vi "PicoScopeospaExampleAWG.vi"() -> ()   [LabVIEW 2010]
uses:
  psospa.dll
panel:
  in  "General AWG Settings":T1={"Peak-to-Peak Voltage"=2.0, "Offset Voltage"=0.0, "Wave Type"=17, "Sweep Type"=0, "Cycles"=10, "Trigger Type"=0, "Trigger Source"=4, "sigGenEnabled"=TRUE, "Trigger Enabled"=FALSE, "autoTriggerPicoSeconds"=0} {"Trigger Source" items=["None"=0, "Scope Trigger"=1, "Software Trigger"=4, "Trigger Raw"=5]; "Trigger Type" items=["Rising", "Falling", "Gate High", "Gate Low"]; "Sweep Type" items=["Up", "Down", "Up-Down", "Down-Up"]; "Wave Type" items=["Sine"=17, "Square"=18, "Triangle"=19, "Ramp Up"=20, "Ramp Down"=21, "Sinc"=22, "Gaussian"=23, "Half Sine"=24, "DC"=1024, "PWM"=4096, "White Noise"=8193, "PRBS"=8194, "Arbitrary"=268435456]; "Offset Voltage" format="%#_6p"; "Peak-to-Peak Voltage" format="%#_6p"}
  in  "Standard Waveform Settings":T2={"(Start) Frequency"=1000.0, "Stop Frequency"=5000.0, "Increment"=1.0, "Dwell Time (seconds)"=0.001, "Sweep Enabled"=FALSE} {"Dwell Time (seconds)" format="%#_6p"; "Stop Frequency" min=0.03 max=1000000.0 format="%#_6p"; "(Start) Frequency" min=0.03 max=1000000.0 format="%#_6p"}
  out "Arbitrary\nWaveform Graph":i16[](graph)
  in  "Duty Cycle":T3={"Use Duty Cycle"=FALSE, "dutyCyclePercent"=20.0}
  in  "Arbitrary Waveform Settings":T4 {"Index Mode" items=["Single", "Dual", "Quad"]}
  out "Device Info":T5={"PICO_DRIVER_VERSION"="ps6000a Windows Driver, 1.0.47.2276", "PICO_USB_VERSION"="2.0", "PICO_HARDWARE_VERSION"="1.1", "PICO_VARIANT_INFO"="6824E", "PICO_BATCH_AND_SERIAL"="FU811/0026", "PICO_CAL_DATE"="06Dec19", "PICO_KERNEL_VERSION"="1.0", "PICO_DIGITAL_HARDWARE_VERSION"="1", "PICO_ANALOGUE_HARDWARE_VERSION"="1", "PICO_FIRMWARE_VERSION_1"="1.7.16.0", "PICO_FIRMWARE_VERSION_2"="1.1.2.0", "PICO_IPP_VERSION"="1.3.0.29", "PICO_DRIVER_PATH"="C:\\Program Files\\Pico Technology\\SDK\\lib\\ps6000a.dll", "PICO_FIRMWARE_VERSION_3"="1.1.49.0", "PICO_FRONT_PANEL_FIRMWARE_VERSION"="0.6.4.0", "Number of Channels"=8, "MSO"=TRUE}
  out "Pico ospa Units":string
  in  "Resolution":u32(ring)=10 items=["8-bit"=0, "12-bit"=1, "14-bit"=2, "15-bit"=3, "16-bit"=4, "10-bit"=10]
  in  "Serial Number":string
  in  "Use Serial Number":bool
  in  "error in (no error)":errorcluster
  in  "Stop S/W \nTrigger":bool
  in  "Apply Settings":bool
  in  "Stop VI":bool
  in  "Software \nTrigger":bool
  # "If Software trigger is selected, press the 'Stop S/W Trigger'\nbutton prior to selecting 'Apply Settings' or 'Stop VI'."
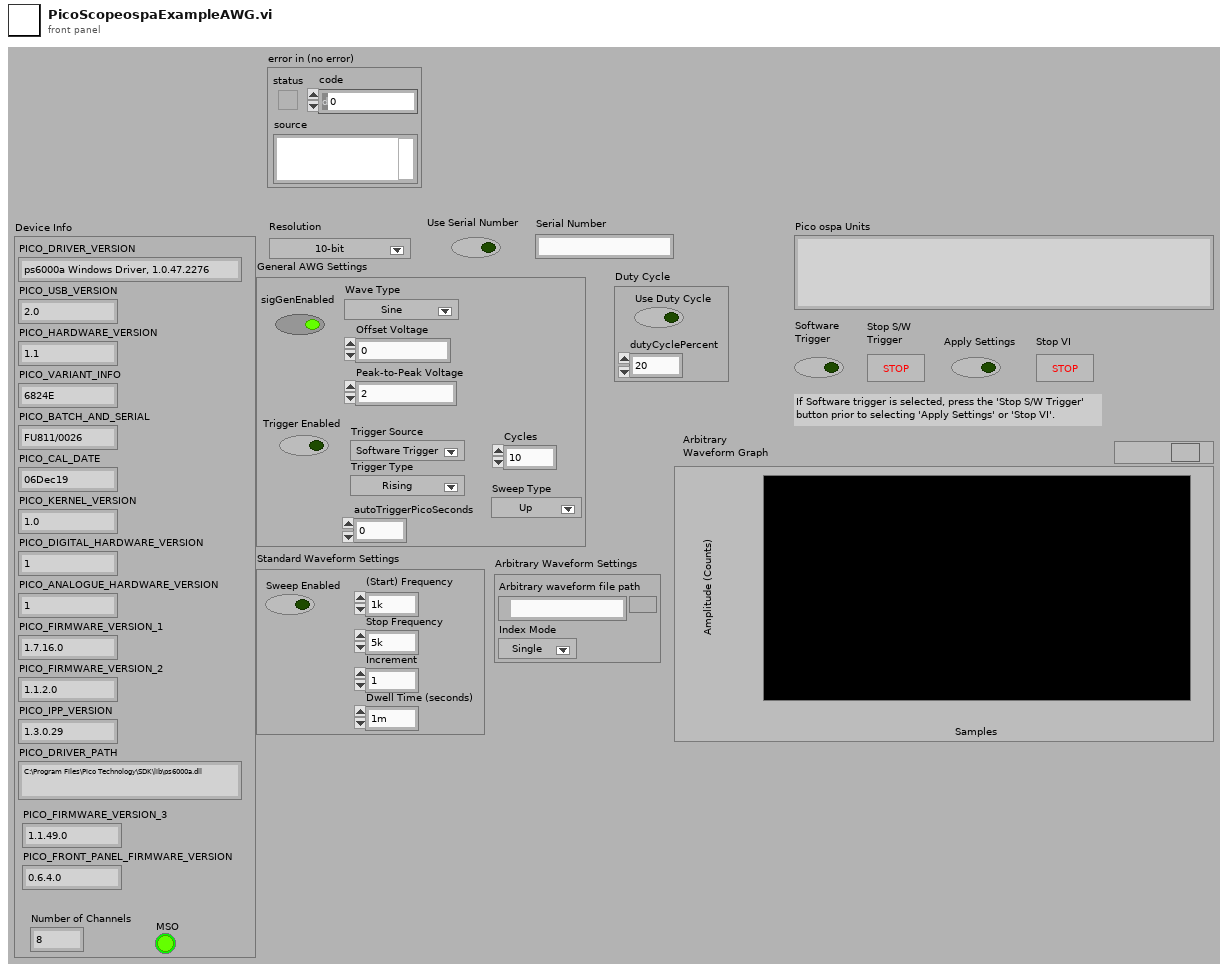
[diagram p1: front panel]
types:
  T1 = cluster{"Peak-to-Peak Voltage":dbl, "Offset Voltage":dbl, "Wave Type":u32, "Sweep Type":u32, "Cycles":u64, "Trigger Type":u32, "Trigger Source":u32, "sigGenEnabled":bool, "Trigger Enabled":bool, "autoTriggerPicoSeconds":u64}
  T2 = cluster{"(Start) Frequency":dbl, "Stop Frequency":dbl, "Increment":dbl, "Dwell Time (seconds)":dbl, "Sweep Enabled":bool}
  T3 = cluster{"Use Duty Cycle":bool, "dutyCyclePercent":dbl}
  T4 = cluster{"Arbirary waveform file path":path, "Index Mode":u32}
  T5 = cluster{"PICO_DRIVER_VERSION":string, "PICO_USB_VERSION":string, "PICO_HARDWARE_VERSION":string, "PICO_VARIANT_INFO":string, "PICO_BATCH_AND_SERIAL":string, "PICO_CAL_DATE":string, "PICO_KERNEL_VERSION":string, "PICO_DIGITAL_HARDWARE_VERSION":string, "PICO_ANALOGUE_HARDWARE_VERSION":string, "PICO_FIRMWARE_VERSION_1":string, "PICO_FIRMWARE_VERSION_2":string, "PICO_IPP_VERSION":string, "PICO_DRIVER_PATH":string, "PICO_FIRMWARE_VERSION_3":string, "PICO_FRONT_PANEL_FIRMWARE_VERSION":string, "Number of Channels":i16, "MSO":bool}
  T6 = cluster{"status":bool, "code":u32, "source":string}
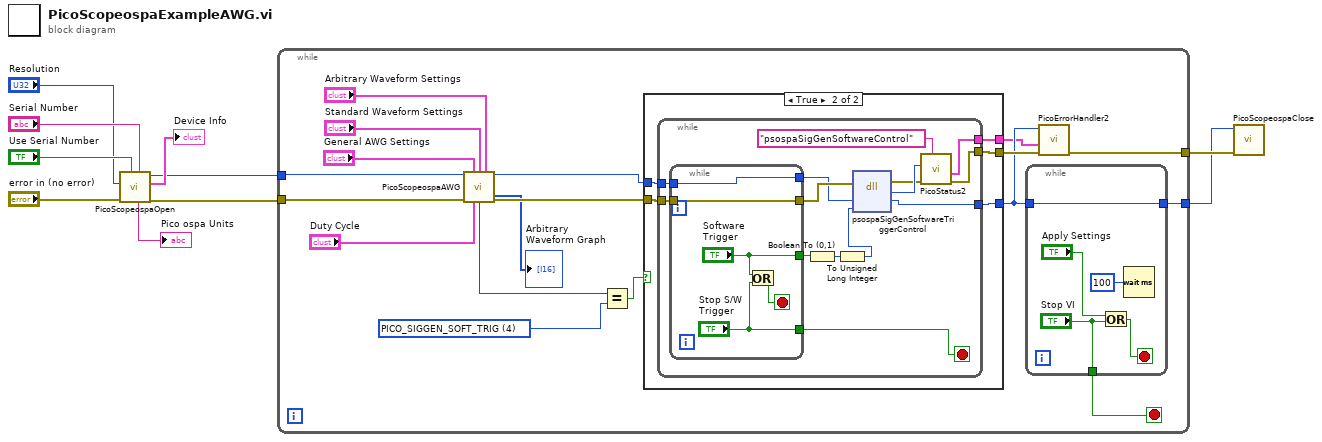
[diagram p0: block diagram]
diagram:
  n1 = call "PicoScopeospaOpen.vi"("Serial Number"="Serial Number", "Use Serial Number"="Use Serial Number", "error in (no error)"="error in (no error)", "Resolution"="Resolution") -> ("error out"=w2:errorcluster, "Device Info"=→"Device Info":T5, "handle out"=w1:i16, "psospa Units"=→"Pico ospa Units":string)  [unwired: 2 in, 2 out]
  n2 = while {
    tunnel: [w25] -> w10
    tunnel: w1 -> [w12]
    tunnel: w2 -> [w23]
    tunnel: [w19] -> w4
    stop <- w27 stop-if-true
    w16 = u32 4 items=["PICO_SIGGEN_SOFT_TRIG"=4]
    n3 = call "PicoScopeospaAWG.vi"("Handle In"=w12, "General AWG Settings"="General AWG Settings", "Standard Waveform Settings"="Standard Waveform Settings", "Arbitrary Waveform Settings"="Arbitrary Waveform Settings", "error in"=w23, "Duty Cycle"="Duty Cycle") -> ("Handle Out"=w22:i16, "Trigger Source Out"=w24:u32, "Arbitrary\nWaveform Graph"=→"Arbitrary\nWaveform Graph":i16[], "error out"=w21:errorcluster)  [unwired: 6 in]
    n4 = Equal?(x=w24, y=w16) -> (x = y?=w28:bool)
    n5 = case shown="True" w28 {
      tunnel: [w35 w38] -> w26
      tunnel: w22 -> [w34 w40]
      tunnel: w21 -> [w35 w39]
      tunnel: [w34 w37] -> w20
      tunnel: [_ w36] -> w11
      frame False {
      }
      frame True {
        n6 = while {
          tunnel: w40 -> [w54]
          tunnel: w39 -> [w53]
          tunnel: [w52] -> w37
          tunnel: [w42] -> w38
          tunnel: [w41] -> w36
          stop <- w50 stop-if-true
          n7 = while {
            tunnel: [w59] -> w48
            tunnel: w54 -> [w59]
            tunnel: ["Software \nTrigger"] -> w51
            tunnel: w53 -> [w58]
            tunnel: [w58] -> w49
            tunnel: ["Stop S/W \nTrigger"] -> w50
            stop <- w55 stop-if-true
            n8 = Or(x="Software \nTrigger", y="Stop S/W \nTrigger") -> (x .or. y?=w55:bool)
          }
          n9 = Boolean To (0,1)(Boolean=w51) -> (0, 1=w47:i16)
          n10 = To Unsigned Long Integer(number=w47) -> (unsigned 32bit integer=w46:u32)
          n11 = dll-call lib="psospa.dll" fn="psospaSigGenSoftwareTriggerControl"(error in=w49, "handle"=w48, "state"=w46) -> (error out=w44:errorcluster, "PICO_STATUS"=w45:u32, "handle"=w52:i16)  [unwired: 3 in, 1 out]
          n12 = call "PicoStatus2.vi"("PICO source"="psospaSigGenSoftwareControl" ("source"), "Error in"=w44, "PICO STATUS"=w45) -> ("error out"=w42:errorcluster, "PICO_STATUS out"=w41:T6)  [unwired: 5 in]
        }
      }
    }
    n13 = while {
      tunnel: ["Stop VI"] -> w27
      tunnel: w20 -> [w30]
      tunnel: [w30] -> w19
      stop <- w33 stop-if-true
      n14 = Or(x="Apply Settings", y="Stop VI") -> (x .or. y?=w33:bool)
      n15 = Wait (ms)(milliseconds to wait=u32 100) -> ()  [unwired: 1 out]
    }
    n16 = call "PicoErrorHandler2.vi"("error in (no error)"=w26, "PICO_STATUS in"=w11, "handle In"=w20) -> ("error out"=w25:errorcluster)  [unwired: 8 in]
  }
  n17 = call "PicoScopeospaClose.vi"("error in (no error)"=w10, "handle in"=w4) -> ()  [unwired: 8 in, 2 out]
